vi "lm35.vi"() -> ()   [LabVIEW 2017]
uses:
  <vilib>/Instr/_visa.llb/VISA Configure Serial Port (Instr).vi
panel:
  out "?":dbl
  out "YÜKSEK DERECE":bool
  out "NORMAL DERECE":bool
  out "DÜÞÜK DERECE":bool
  in  "YÜKSEK DERECE":dbl
  in  "NORMAL DERECE":dbl
  in  "Stop Button":bool
  out "TEMPERATURE":dbl(knob) scale=0.0..150.0
  in  "Port COM":refnum<visa-resource-name>
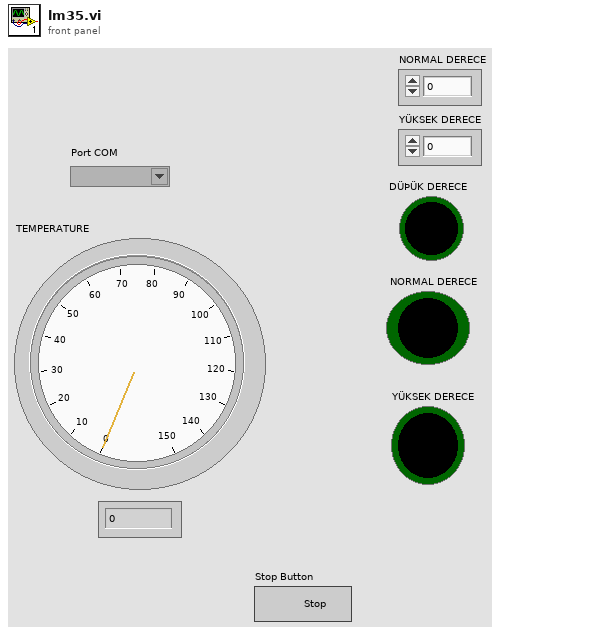
[diagram p1: front panel]
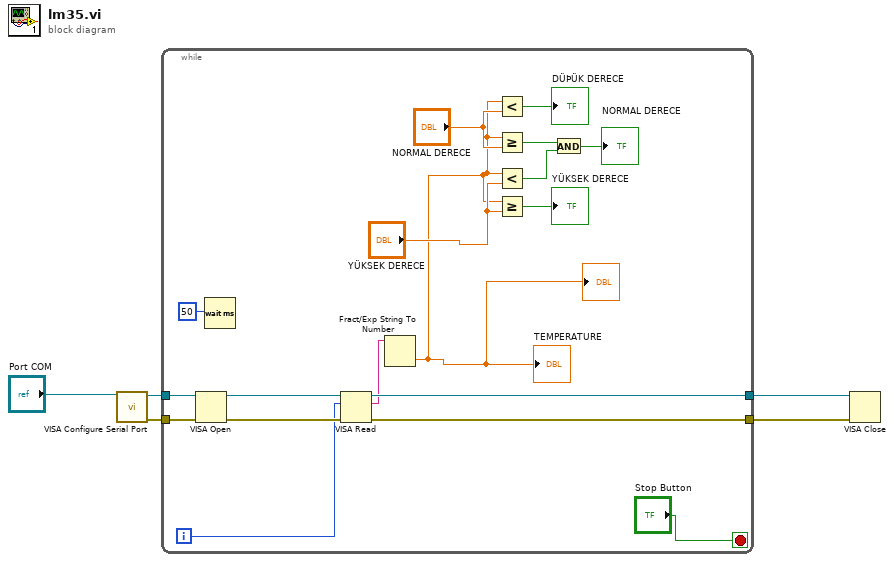
[diagram p0: block diagram]
diagram:
  n1 = call-poly "VISA Configure Serial Port"("VISA resource name"="Port COM") -> ("VISA resource name out"=w2:refnum<visa-resource-name>, "error out"=w5:errorcluster)  [unwired: 13 in]
  n2 = while {
    tunnel: w5 -> [w23]
    tunnel: [w21] -> w4
    tunnel: [w20] -> w3
    tunnel: w2 -> [w18]
    i -> [w17]
    stop <- "Stop Button" stop-if-true
    n3 = VISA Open(error in (no error)=w23, VISA resource name=w18) -> (VISA resource name=w19:refnum<visa-resource-name>, error out=w22:errorcluster)  [unwired: 3 in]
    n4 = Wait (ms)(milliseconds to wait=u32 50 ("millisecond timer value")) -> ()  [unwired: 1 out]
    n5 = VISA Read(VISA resource name=w19, byte count=w17, error in (no error)=w22) -> (VISA resource name out=w20:refnum<visa-resource-name>, read buffer=w15:string, error out=w21:errorcluster)  [unwired: 1 out]
    n6 = Fract/Exp String To Number(string=w15) -> (number=w6:dbl)  [unwired: 3 in, 1 out]
    "TEMPERATURE" <- w6
    "?" <- w6
    n7 = Less?(x=w6, y="NORMAL DERECE") -> (x < y?=→"DÜÞÜK DERECE":bool)
    n8 = Greater Or Equal?(x=w6, y="NORMAL DERECE") -> (x >= y?=w12:bool)
    n9 = Less?(x=w6, y="YÜKSEK DERECE") -> (x < y?=w11:bool)
    n10 = Greater Or Equal?(x=w6, y="YÜKSEK DERECE") -> (x >= y?=→"YÜKSEK DERECE":bool)
    n11 = And(x=w12, y=w11) -> (x .and. y?=→"NORMAL DERECE":bool)
  }
  n12 = VISA Close(VISA resource name=w3, error in (no error)=w4) -> ()  [unwired: 1 out]
